vi "Draw Single Expanded Terminal.vi"(7 "Expanded Index":i32, 8 "Value Index":i32, 9 "State":T1={"Worker Library Path"=path "", "Block Label"="", "Types"=[], "Selections"=[], "Icon"={"image type"=0, "image depth"=0, "image"=[], "mask"=[], "colors"=[], "Rectangle"={"left"=0, "top"=0, "right"=0, "bottom"=0}}, "Errors"={"Terminals"=[], "Generate"={"status"=FALSE, "code"=0, "source"=""}, "General"={"status"=FALSE, "code"=0, "source"=""}}, "Calculated Sizes"={"Block Width"=0, "Block Height"=0, "Half Width"=0, "Icon Top"=0, "Icon Bottom"=0, "Label Width"=0, "Half Label"=0, "Label Top"=0, "Text Width"=0, "Half Text"=0, "Text Height"=0, "Label Height"=0, "Expanded Width"=0, "Label Bottom"=0, "Expanded Top"=0, "Expanded Bottom"=0, "Expanded Height"=0, "Min Height"=0, "Max Height"=0}, "Special Terminal Indices"={"Action"=-1, "Init"=-1, "Tag"=-1, "State in"=-1, "State out"=-1, "Error"=-1, "Control"=-1, "Config"=-1}, "Terminals"=[], "Temp VI Name"="", "Description"="", "Smol Mode"=FALSE}, 11 "Picture In":picture) -> (3 "Picture":picture)   [LabVIEW 2022 SP3, in "FlexBlocks Support.lvlib"]
uses:
  FlexBlocks Support.lvlib
  Flex Block/State.ctl
  Type Descriptor.ctl
  Terminal Direction.ctl
  Value Mode.ctl
  Special Terminal.ctl
  <vilib>/picture/picture.llb/imagedata.ctl
  XNode Errors.ctl
  Calculated Sizes.ctl
  Special Terminal Indices.ctl
  Terminal Status.ctl
  Terminal State.ctl
  Terminal Draw Style.ctl
  Flex Block/Flex Block.xnode
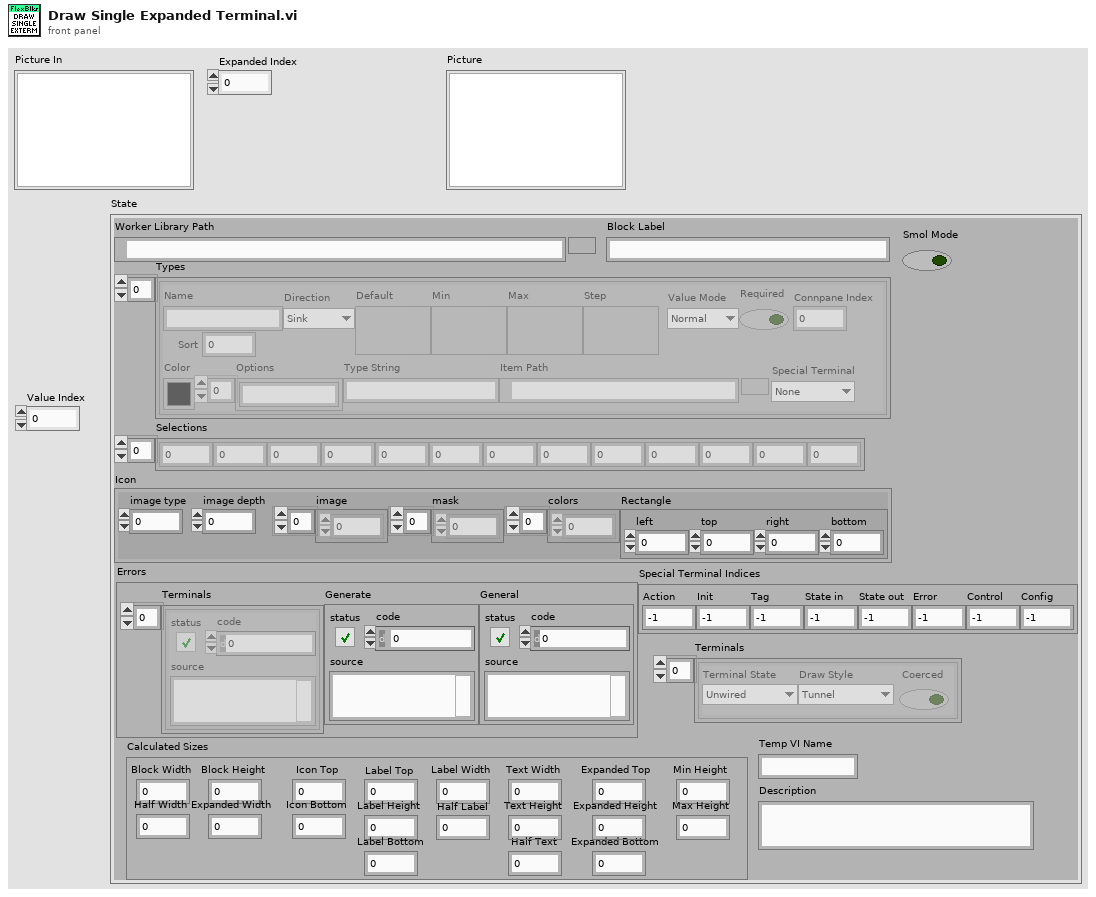
[diagram p1: front panel]
types:
  T1 = typedef "Flex Block.xnode/State.ctl" = cluster{"Worker Library Path":path, "Block Label":string, "Types":T2[], "Selections":i32[], "Icon":T6, "Errors":T7, "Calculated Sizes":T8, "Special Terminal Indices":T9, "Terminals":T10[], "Temp VI Name":string, "Description":string, "Smol Mode":bool}
  T2 = typedef "FlexBlocks Support.lvlib/Type Descriptor.ctl" = cluster{"Name":string, "Direction":T3, "Default":variant, "Min":variant, "Max":variant, "Step":variant, "Value Mode":T4, "Color":u32, "Options":string[], "Type String":string, "Item Path":path, "Required":bool, "Connpane Index":i32, "Special Terminal":T5, "Sort":i32}
  T3 = typedef "FlexBlocks Support.lvlib/Terminal Direction.ctl" = enum16{"Sink", "Source"}
  T4 = typedef "FlexBlocks Support.lvlib/Value Mode.ctl" = enum16{"Normal", "Range", "Select"}
  T5 = typedef "FlexBlocks Support.lvlib/Special Terminal.ctl" = enum16{"None", "Action", "Init", "Tag", "State in", "State out", "Error", "Control", "Config"}
  T6 = typedef "imagedata.ctl" = cluster{"image type":i32, "image depth":i32, "image":u8[], "mask":u8[], "colors":u32[], "Rectangle":cluster{"left":i16, "top":i16, "right":i16, "bottom":i16}}
  T7 = typedef "FlexBlocks Support.lvlib/XNode Errors.ctl" = cluster{"Terminals":errorcluster[], "Generate":errorcluster, "General":errorcluster}
  T8 = typedef "FlexBlocks Support.lvlib/Calculated Sizes.ctl" = cluster{"Block Width":i32, "Block Height":i32, "Half Width":i32, "Icon Top":i32, "Icon Bottom":i32, "Label Width":i32, "Half Label":i32, "Label Top":i32, "Text Width":i32, "Half Text":i32, "Text Height":i32, "Label Height":i32, "Expanded Width":i32, "Label Bottom":i32, "Expanded Top":i32, "Expanded Bottom":i32, "Expanded Height":i32, "Min Height":i32, "Max Height":i32}
  T9 = typedef "FlexBlocks Support.lvlib/Special Terminal Indices.ctl" = cluster{"Action":i32, "Init":i32, "Tag":i32, "State in":i32, "State out":i32, "Error":i32, "Control":i32, "Config":i32}
  T10 = typedef "FlexBlocks Support.lvlib/Terminal Status.ctl" = cluster{"Terminal State":T11, "Draw Style":T12, "Coerced":bool}
  T11 = typedef "FlexBlocks Support.lvlib/Terminal State.ctl" = enum16{"Unwired", "BadType", "BadRef", "Channel", "Value", "Control Ref"}
  T12 = typedef "FlexBlocks Support.lvlib/Terminal Draw Style.ctl" = enum16{"Tunnel", "BadType", "BadRef", "Channel", "Value", "Control Ref"}
  T13 = cluster{"left":i16, "top":i16, "right":i16, "bottom":i16}
  T14 = typedef "FlexBlocks Support.lvlib/Size Constants.ctl" = cluster{"Icon Size":i32, "Name H Pad":i32, "Name V Pad":i32, "Max Label Width":i32, "Value Width":i32, "Frame Padding":i32, "Vertical Margin":i32, "Min Width":i32, "Min Height":i32, "Collapsed Spacing":i32, "Terminal Center Offset":i32}
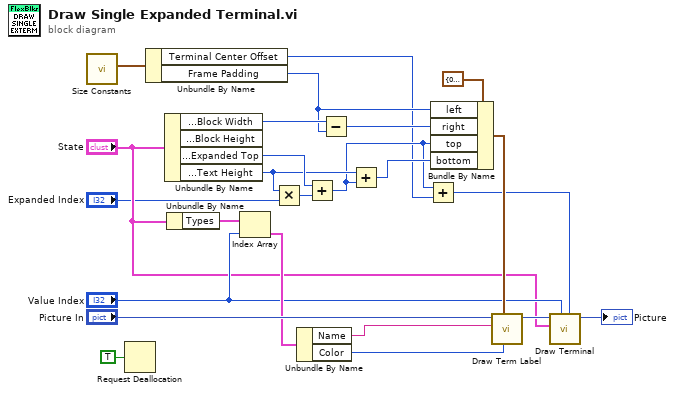
[diagram p0: block diagram]
diagram:
  n1 = call "Size Constants.vi"() -> ("Size Constants"=w16:T14)  [unwired: 11 in]
  n2 = Request Deallocation(TRUE ("flag")) -> ()
  n3 = Unbundle By Name(w16) -> ("Terminal Center Offset"=w6:i32, "Frame Padding"=w10:i32)
  n4 = Unbundle By Name("State") -> ("Calculated Sizes.Block Width"=w14:i32, "Calculated Sizes.Expanded Top"=w20:i32, "Calculated Sizes.Text Height"=w13:i32)  [unwired: 1 out]
  n5 = Unbundle By Name("State") -> ("Types"=w22:T2[])
  n6 = Index Array(array=w22, index="Value Index") -> (element=w21:T2)
  n7 = Multiply(x=w13, y="Expanded Index") -> (x*y=w19:i32)
  n8 = Unbundle By Name(w21) -> ("Name"=w23:string, "Color"=w3:u32)
  n9 = Add(x=w20, y=w19) -> (x+y=w7:i32)
  n10 = Subtract(x=w14, y=w10) -> (x-y=w15:i32)
  n11 = Add(x=w13, y=w7) -> (x+y=w12:i32)
  n12 = Add(x=w7, y=w6) -> (x+y=w5:i32)
  n13 = Bundle By Name(cluster=T13 {"left"=0, "top"=0, "right"=150, "bottom"=100} ("Bounds"), "left"=w10, "right"=w15, "top"=w7, "bottom"=w12) -> (w17:T13)
  n14 = call "Draw Term Label.vi"("Type Color"=w3, "Bounds"=w17, "Name"=w23, "Picture In"="Picture In") -> ("Picture"=w9:picture)  [unwired: 7 in]
  n15 = call "Draw Terminal.vi"("Center"=w5, "Value Index"="Value Index", "State"="State", "Picture In"=w9) -> ("Picture"=→"Picture":picture)  [unwired: 7 in]
